vi "Description with Channel Prefix.vi"(6 "error in":errorcluster, 8 "Description":string, 9 "channel":i32) -> (0 "error out":errorcluster, 2 "Step Name":string, 3 "Test Name":string)   [LabVIEW 2010]
doc: "This function inserts the Channel Number into the Measurement Name field of a CDT cluster."
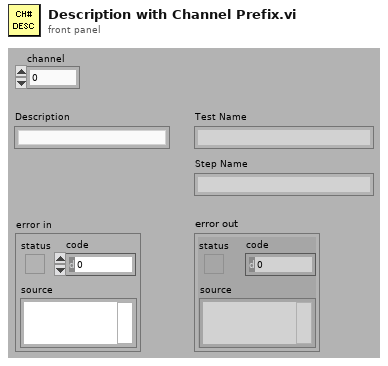
[diagram p1: front panel]
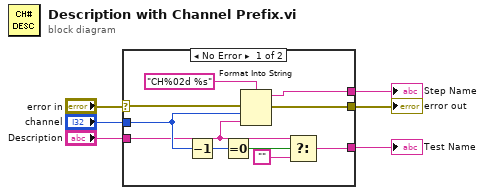
[diagram p0: block diagram]
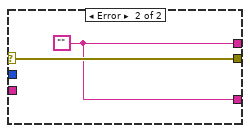
[diagram p2: hidden frame]
diagram:
  n1 = case shown="No Error" "error in" {
    selector: "error in" -> [w14 w18]
    tunnel: [w15 w18] -> w6
    tunnel: "channel" -> [w12 _]
    tunnel: [w11 w17] -> w3
    tunnel: [w10 w17] -> w2
    tunnel: "Description" -> [w8 _]
    frame No Error {
      n2 = Decrement(x=w12) -> (x-1=w7:i32)
      n3 = Equal To 0?(x=w7) -> (x = 0?=w13:bool)
      n4 = Format Into String(format string="CH%02d %s", error in=w14, w12, w8) -> (resulting string=w10:string, error out=w15:errorcluster)  [unwired: 1 in]
      n5 = Select(t=w8, s=w13, f="") -> (s? t:f=w11:string)
    }
    frame Error {
      w17 = ""
    }
  }
  "error out" <- w6
  "Step Name" <- w2
  "Test Name" <- w3
